vi "TestGraph.vi"() -> ()   [LabVIEW 2013]
uses:
  <vilib>/Utility/file.llb/Read From Spreadsheet File (string).vi
panel:
  out "élément":string
  out "Graphe déroulant":waveform(dbl)(graph)
  out "Graphe":waveform(dbl)(graph)
  out "Tableau":dbl[][](array[numeric])
  out "Col_Hygrometrie":i32=4
  out "Col_Temperature":i32=4
  out "Col_Arrosage":i32=4
  out "Col_Date":i32=4
  out "Col_TS":i32=4
  out "Col_Compo":i32=4
  out "Col_Chauffage":i32=4
  out "Col_Ventillation":i32=4
  out "Col_Mode":i32=4
  out "Col_Level":i32=4
  in  "entrée d'erreur":errorcluster
  in  "chemin du fichier (utiliser une boîte de dialogue)":path
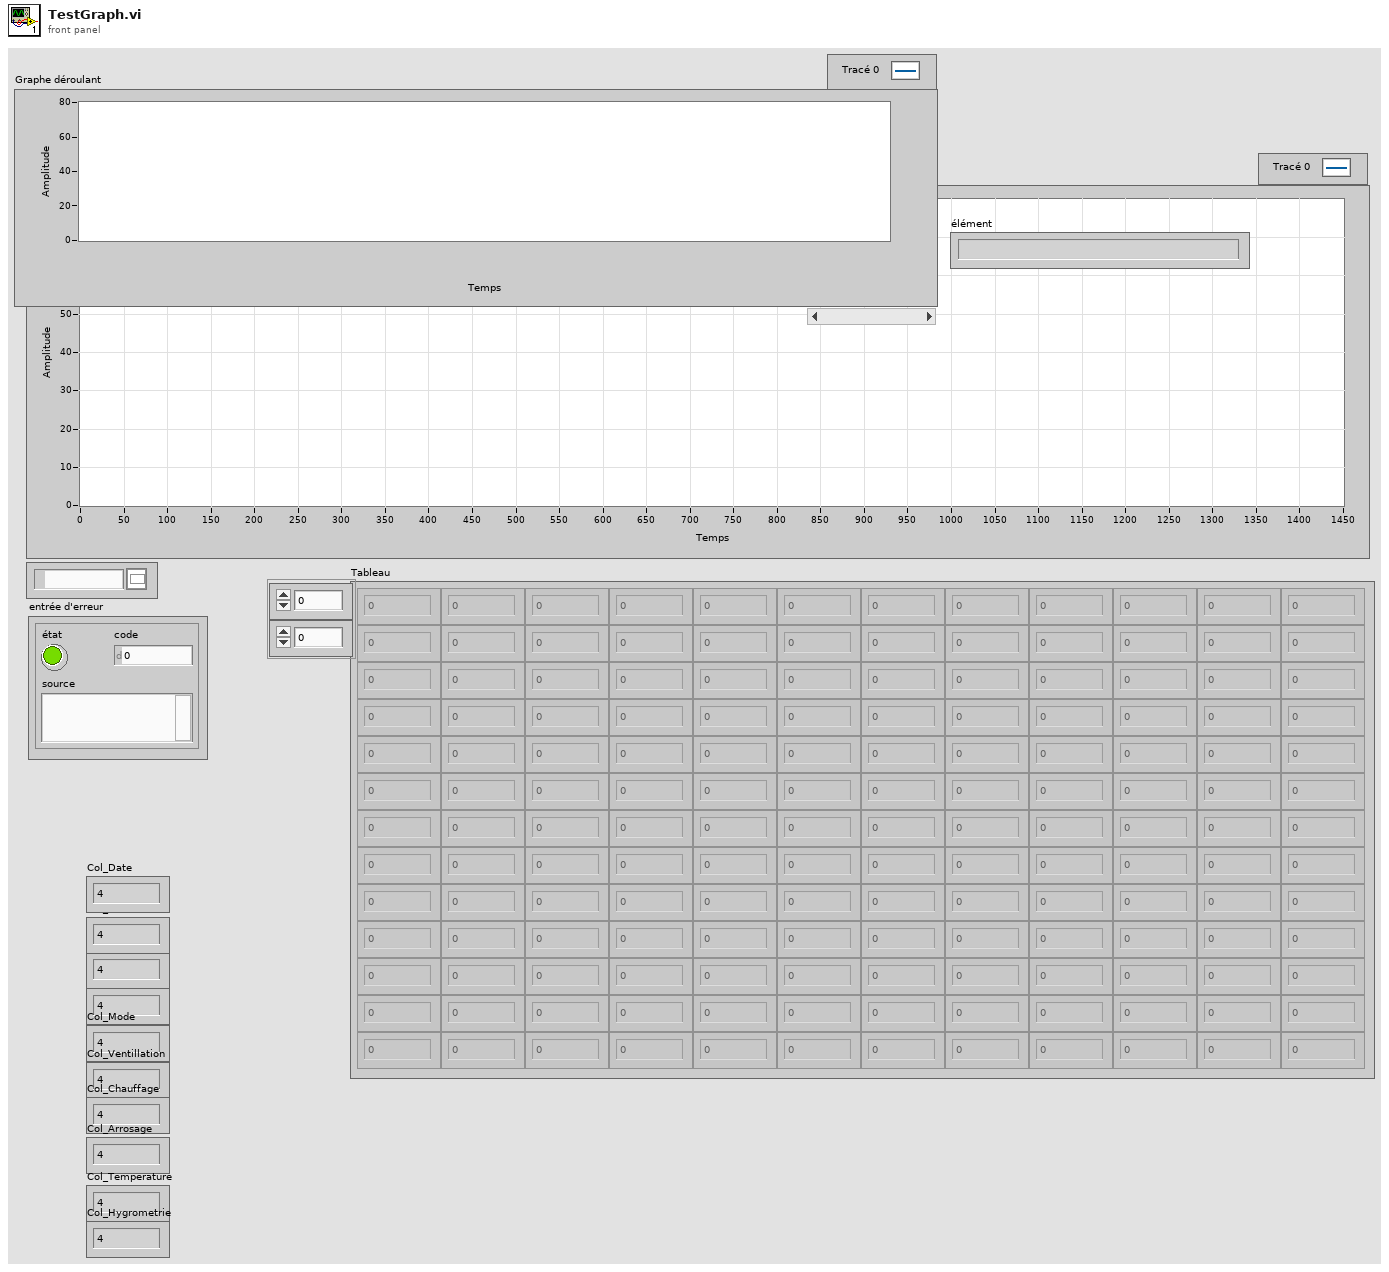
[diagram p1: front panel]
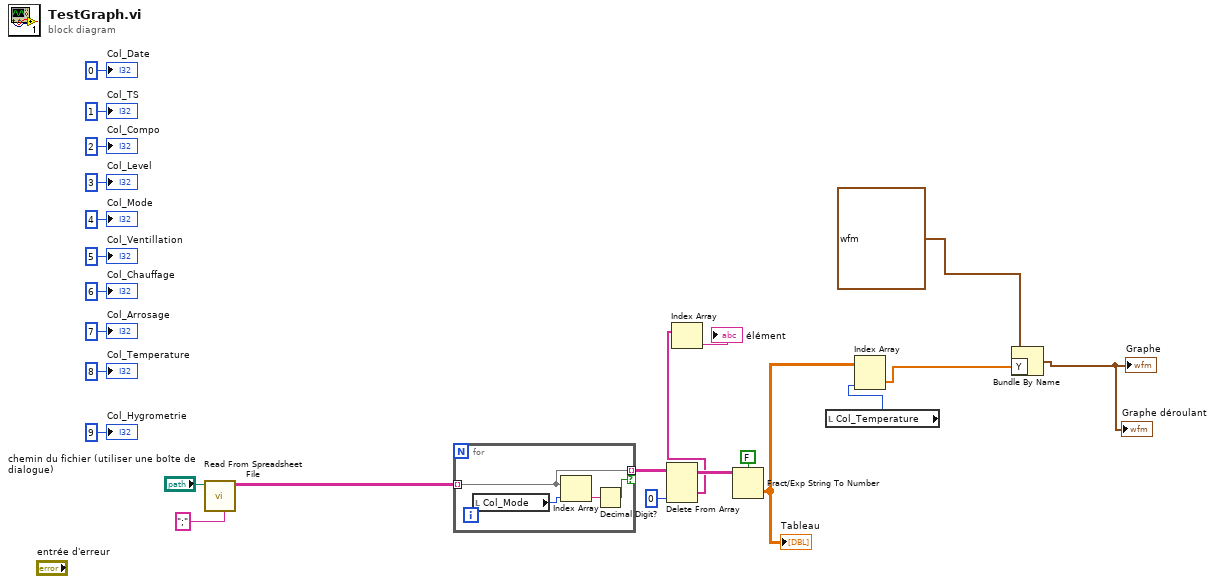
[diagram p0: block diagram]
diagram:
  n1 = call-poly <vilib>:"Read From Spreadsheet File.vi"("delimiter (\\t)"=";" ("delimiter (\\t)"), "file path (dialog if empty)"="chemin du fichier (utiliser une boîte de dialogue)") -> ("all rows"=w22:string[][])  [unwired: 5 in, 4 out]
  n2 = for {
    tunnel: w22 -> [w27] mode=indexing
    tunnel: [w27] -> w3 mode=indexing if=w26
    n3 = local read "Col_Mode"() -> (w25:i32)
    n4 = Index Array(array=w27, index=w25) -> (element=w28:string)
    n5 = Decimal Digit?(1:w28) -> (0:w26:bool)
  }
  n6 = Delete From Array(array=w3, index (col)=0 ("indice désactivé (col)")) -> (deleted portion=w2:string[], array with subset deleted=w10:string[][])  [unwired: 2 in]
  n7 = Index Array(array=w2) -> (element=→"élément":string)  [unwired: 1 in]
  n8 = Fract/Exp String To Number(use system decimal point (T)=FALSE ("utiliser le séparateur décimal du système (V)"), string=w10) -> (number=w7:dbl[][])  [unwired: 2 in, 1 out]
  "Tableau" <- w7
  n9 = local read "Col_Temperature"() -> (w6:i32)
  n10 = Index Array(array=w7, index (col)=w6) -> (element=w5:dbl[])  [unwired: 1 in]
  n11 = Bundle By Name(cluster=waveform(dbl) {"t0"=timestamp(0 s since 1904-01-01), "dt"=1.0, "Y"=[]} ("waveform"), "Y"=w5) -> (→"Graphe" →"Graphe déroulant":waveform(dbl))
  "Col_Level" <- 3 ("indice")
  "Col_Mode" <- 4 ("indice")
  "Col_Ventillation" <- 5 ("indice")
  "Col_Chauffage" <- 6 ("indice")
  "Col_Compo" <- 2 ("indice")
  "Col_TS" <- 1 ("indice")
  "Col_Date" <- 0 ("indice")
  "Col_Arrosage" <- 7 ("indice")
  "Col_Temperature" <- 8 ("indice")
  "Col_Hygrometrie" <- 9 ("indice")
